vi "RT Driver VI.vi"(6 "Device Clock":string, 9 "Device Inputs FIFO":refnum<k33>, 10 "Device Outputs FIFO":refnum<k33>, 11 "Device Reference":T1 format="%.0x") -> ()   [LabVIEW 2015, in "Engine Simulation Toolkit Engine.lvlib"]
uses:
  Engine Simulation Toolkit Engine.lvlib
  <vilib>/NI Veristand/Custom Device API/Custom Device Item Ref.ctl
  <vilib>/Platform/TimedLoop/XDataNode/timing_clust.ctl
  <vilib>/Platform/TimedLoop/XDataNode/nitl_modes.ctl
  <vilib>/Platform/TimedLoop/XDataNode/wakeup.ctl
  Digital Pattern Gen 1.0 In Place Input Write Structure.vi
  APU 1.0 In Place Input Write Structure.vi
  APU 1.0 In Place Output Read Structure.vi
  Analog Replay 1.0 In Place Input Write Structure.vi
  Knock Cylinder 1.0 In Place Input Write Structure.vi
  Knock Sensor 1.0 In Place Input Write Structure.vi
  Directional Speed 1.0 In Place Input Write Structure.vi
  APU 1.1 In Place Input Write Structure.vi
  APU 1.1 In Place Output Read Structure.vi
  Digital Pattern Gen 1.3 In Place Input Write Structure.vi
  Digital Pattern Gen 1.3 In Place Settings Write Structure.vi
  APU 1.3 In Place Input Write Structure.vi
  APU 1.3 In Place Output Read Structure.vi
  Digital Pattern Gen 1.0 Write Inputs.vi
  APU 1.0 Write Inputs.vi
  Analog Replay 1.0 Voltage Scaling.vi
  Knock Cylinder 1.0 Write Inputs.vi
  Knock Sensor 1.0 Write Inputs.vi
  Directional Speed 1.0 Write Inputs.vi
  Digital Pattern Gen 1.3 Write Inputs.vi
  Digital Pattern Gen 1.3 Tooth to Edges.vi
  Shared/Angle in degrees to u16.vi
  Digital Pattern Gen 1.3 Validate Fault Positions.vi
  Shared/DBL Speed to FXP.vi
  Shared/Probability % to compare.vi
  Analog Replay 1.0 FPGA Inputs Write Node.vi
  Digital Pattern Gen 1.3 FPGA Settings Write Node.vi
  Digital Pattern Gen 1.0 FPGA Inputs Write Node.vi
  Knock Sensor 1.0 FPGA Inputs Write Node.vi
  Knock Cylinder 1.0 FPGA Inputs Write Node.vi
  Directional Speed 1.0 FPGA Inputs Write Node.vi
  Event Timing Capture 1.0 In Place Output Read Structure.vi
  Event Timing Measure 1.1 In Place Output Read Structure.vi
  Event Timing Measure 1.0 In Place Output Read Structure.vi
  APU 1.0 Read Outputs.vi
  APU 1.0 FPGA Inputs Write Node.vi
  <vilib>/Platform/TimedLoop/XDataNode/XDataNode.xnode
  <vilib>/NI Veristand/Custom Device Tools/Custom Device Utility Library/Custom Device Utility Library.lvlib
  <vilib>/Platform/TimedLoop/XDataNode/XDNodeRunTimeDep.lvlib
  <vilib>/NI Veristand/Custom Device API/Custom Device API.lvlib
panel:
  in  "Initialization Status Notifier":refnum<notifier>
  in  "Status Notifier":refnum<notifier>
  # "Custom Device Template\nv1.0"
  # "Use this template as a starting point for creating a custom device code module. The input controls shown here are specially named controls that the system will use to provide the device loop with data. The controls are not required for the device loop to run. For instance, if the device doesn't produce any output data, then you don't need the Device Outputs FIFO control. If you do use these controls, however, they need to have these exact names to be functional."
  # "The optional status notifier element is used to notify the RT engine of the last state of the custom device, and to indicate the device has completed execution. If this control is not used, a default No Error value is returned to the system when the device finishes execution.\n\nNote: This error state is not checked until the system shuts down. Use an output status channel to send more immediate status values to the system."
  # "This optional input can be used to send the VeriStand Engine the final status of the custom device initalization process. If this control exists on the custom device front panel, the VeriStand Engine will wait for a status update before starting up. If the custom device reports an error, that will abort the execution of the current configuration in the VeriStand Engine.\n\nThis control can be deleted if the custom device does not need to send the initialization status update."
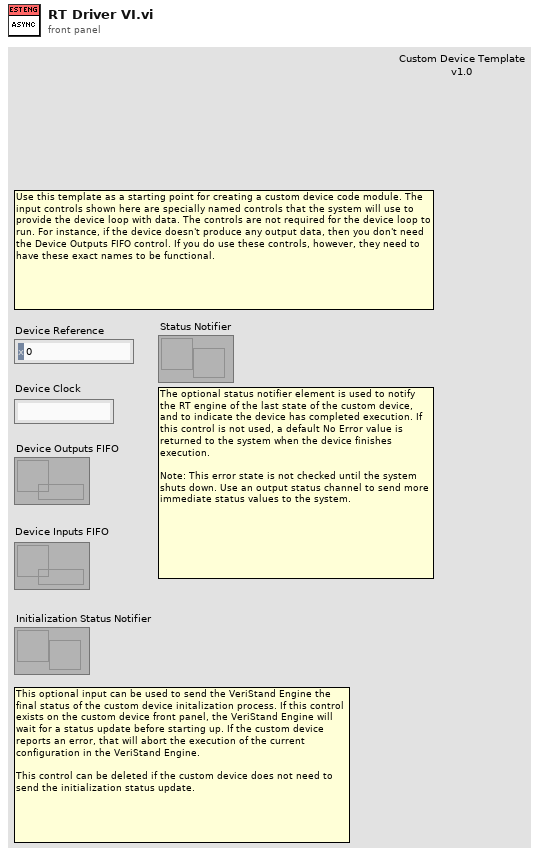
[diagram p1: front panel]
types:
  T1 = typedef "Custom Device API.lvlib/Custom Device Item Ref.ctl" = u64
  T2 = typedef "Engine Simulation Toolkit Engine.lvlib/RT Data.ctl" = cluster{"Compiled Data":T3, "FPGA Refs":T28}
  T3 = typedef "Engine Simulation Toolkit Shared.lvlib/Compiled Data.ctl" = cluster{"Init":T4, "1.0 APUs":T5[], "Status":T7, "DevOutFIFO":refnum<k33>, "DevInFIFO":refnum<k33>, "Device Inputs":dbl[], "Device Outputs":dbl[], "Last Device Inputs":dbl[], "1.0 Analog Replays":T8[], "Unused Analog Replays":string[], "1.0 Digital Pattern Gens":T10[], "Unused Digital Pattern Gens":string[], "1.0 Event Captures":T12[], "1.0 Event Measures":T14[], "1.0 Knock Sensors":T16[], "1.0 Knock Cylinders":T18[], "1.0 Directional Speed":T20[], "Unused Directional Sensors":string[], "1.1 APUs":T22[], "1.1 Event Measures":T23[], "1.3 Digital Pattern Gens":T24[], "Bitfile EST Version":T26, "1.3 APUs":T27[]}
  T4 = typedef "Engine Simulation Toolkit Shared.lvlib/Engine Init Data.ctl" = cluster{"CPU":i32, "RIO Address":string, "Decimation":i64, "Priority":i32, "Name":string, "Bitfile Path":path, "Input FIFO Size":i32, "Output FIFO Size":i32}
  T5 = typedef "Engine Simulation Toolkit Shared.lvlib/1.0 APU Engine Data.ctl" = cluster{"register names":cluster{"shared settings":string, "input":string, "settings":string, "output":string}, "shared settings":cluster{"cycle start":fxp<+,2,2>, "crank start":u16, "stuck limit":fxp<+,18,18>}, "settings":cluster{"acceleration":fxp<+,18,-20>, "max cycle":fxp<+,2,2>, "enable accel":bool}, "FIFO indexes":T6, "input":cluster{"desired speed":fxp<+/-,23,2>, "reset":bool}, "degrees of 1 cycle u16":dbl, "degrees of 1 crank u16":dbl}
  T6 = typedef "Engine Simulation Toolkit Shared.lvlib/1.0 APU Engine FIFO Idxs.ctl" = cluster{"inputs":cluster{"desired speed":i32, "reset":i32}, "outputs":cluster{"crank angle":i32, "cycle angle":i32, "actual speed":i32}}
  T7 = typedef "Engine Simulation Toolkit Shared.lvlib/Engine Status Data.ctl" = cluster{"FIFO indexes":cluster{"code":i32, "loop duration":i32, "late count":i32}}
  T8 = typedef "Engine Simulation Toolkit Shared.lvlib/1.0 Analog Replay Engine Data.ctl" = cluster{"register names":cluster{"load input":string, "settings":string, "input":string}, "settings":cluster{"ReverseNegate":bool, "CycleAngle":bool, "SpeedThreshold":fxp<+/-,23,2>, "AOBelowThreshold":i16}, "FIFO indexes":T9, "input":cluster{"Offset":i16, "VScaleSlope":fxp<+,18,6>, "VScaleIntercept":fxp<+/-,18,3>}, "offset convert":dbl, "DAC LUT":i16[], "SE_VScaleIntercept":fxp<+/-,18,3>, "SE_VScaleSlope":fxp<+,18,6>, "VOverride":bool, "ResetVolts":bool}
  T9 = typedef "Engine Simulation Toolkit Shared.lvlib/1.0 Analog Replay FIFO Idxs.ctl" = cluster{"enable voltage":i32, "volt slope":i32, "volt intercept":i32, "offset":i32}
  T10 = typedef "Engine Simulation Toolkit Shared.lvlib/1.0 Digital Pattern Gen Engine Data.ctl" = cluster{"register names":cluster{"load input":string, "settings":string, "input":string}, "settings":cluster{"edge 1":u16, "edge 2":u16, "cycle angle":bool, "enabled":bool, "first falling":bool}, "FIFO indexes":T11, "input":cluster{"Offset":i16}, "offset convert":dbl, "Position LUT":u16[]}
  T11 = typedef "Engine Simulation Toolkit Shared.lvlib/1.0 Digital Pattern Gen FIFO Idxs.ctl" = cluster{"offset":i32}
  T12 = typedef "Engine Simulation Toolkit Shared.lvlib/1.0 Event Timing Capture Engine Data.ctl" = cluster{"register names":cluster{"output":string}, "FIFO indexes":T13, "degrees of 1 u16":dbl, "wrap":bool, "window min":u16, "duration convert":dbl, "default start":dbl, "default end":dbl, "ref angle":dbl}
  T13 = typedef "Engine Simulation Toolkit Shared.lvlib/1.0 Event Timing Capture FIFO Idxs.ctl" = cluster{"start angle":i32, "end angle":i32, "duration":i32}
  T14 = typedef "Engine Simulation Toolkit Shared.lvlib/1.0 Event Timing Measure Engine Data.ctl" = cluster{"register names":cluster{"settings":string, "output":string}, "settings":cluster{"max":u16, "min":u16, "active high":bool, "wrap":bool, "full window":bool}, "FIFO indexes":T15}
  T15 = typedef "Engine Simulation Toolkit Shared.lvlib/1.0 Event Timing Measure FIFO Idxs.ctl" = cluster{"stuck active":i32, "win all active":i32, "win orph start":i32, "win orph end":i32}
  T16 = typedef "Engine Simulation Toolkit Shared.lvlib/1.0 Knock Sensor Engine Data.ctl" = cluster{"register names":cluster{"settings":string, "input":string}, "settings":cluster{"low freq (periods/tick)":fxp<+,32,0>, "high freq (periods/tick)":fxp<+,32,0>, "duration (1.25MHz tics)":fxp<+,18,18>, "low freq speed slope":fxp<+,16,-3>, "low freq speed intercept":fxp<+,10,-10>, "low freq by speed":bool}, "DAC multiplier":dbl, "FIFO indexes":T17, "input":cluster{"low freq scaler":fxp<+,10,0>}}
  T17 = typedef "Engine Simulation Toolkit Shared.lvlib/1.0 Knock Sensor FIFO Idxs.ctl" = cluster{"amp":i32}
  T18 = typedef "Engine Simulation Toolkit Shared.lvlib/1.0 Knock Cylinder Engine Data.ctl" = cluster{"register names":cluster{"settings":string, "input":string}, "settings":cluster{"seed":u16, "reset":bool}, "input":cluster{"probability compare":u16, "high freq scaler":fxp<+,10,0>, "trigger position":u16}, "DAC multiplier":dbl, "FIFO indexes":T19, "Angle multiplier":dbl}
  T19 = typedef "Engine Simulation Toolkit Shared.lvlib/1.0 Knock Cylinder FIFO Idxs.ctl" = cluster{"prob":i32, "amp":i32, "pos":i32}
  T20 = typedef "Engine Simulation Toolkit Shared.lvlib/1.0 Directional Speed Engine Data.ctl" = cluster{"register names":cluster{"settings":string, "input":string, "load input":string}, "settings":cluster{"Upper Value":u16, "Lower Value":u16, "Upper Index":fxp<+,10,10>, "Lower Index":fxp<+,10,10>, "Enabled":bool}, "input":cluster{"td (tics)":u16, "tf (tics)":u16, "tr (tics)":u16}, "FIFO indexes":T21, "Tooth Centers LUT":u16[]}
  T21 = typedef "Engine Simulation Toolkit Shared.lvlib/1.0 Directional Speed FIFO Idxs.ctl" = cluster{"td":i32, "tf":i32, "tr":i32}
  T22 = typedef "Engine Simulation Toolkit Shared.lvlib/1.1 APU Engine Data.ctl" = cluster{"register names":cluster{"shared settings":string, "input":string, "settings":string, "output":string, "go":string}, "shared settings":cluster{"cycle start":fxp<+,2,2>, "crank start":u16, "stuck limit":fxp<+,18,18>}, "settings":cluster{"acceleration":fxp<+,18,-20>, "max cycle":fxp<+,2,2>, "enable accel":bool}, "FIFO indexes":T6, "input":cluster{"desired speed":fxp<+/-,23,2>, "reset":bool}, "degrees of 1 cycle u16":dbl, "degrees of 1 crank u16":dbl}
  T23 = typedef "Engine Simulation Toolkit Shared.lvlib/1.1 Event Timing Measure Engine Data.ctl" = cluster{"register names":cluster{"settings":string, "output":string}, "settings":cluster{"max":u16, "min":u16, "active high":bool, "wrap":bool}, "FIFO indexes":T15}
  T24 = typedef "Engine Simulation Toolkit Shared.lvlib/1.3 Digital Pattern Gen Engine Data.ctl" = cluster{"register names":cluster{"load input":string, "settings":string, "input":string}, "settings":cluster{"edge 1":u16, "edge 2":u16, "cycle angle":bool, "enabled":bool, "first falling":bool, "fault":bool, "fault wrap":bool, "fault value":bool, "fault count":fxp<+,4,4>, "use fault count":bool}, "FIFO indexes":T25, "input":cluster{"Offset":i16}, "deg to u16 scale":dbl, "Position LUT":u16[], "# of teeth":i16, "max angle":dbl}
  T25 = typedef "Engine Simulation Toolkit Shared.lvlib/1.3 Digital Pattern Gen FIFO Idxs.ctl" = cluster{"offset":i32, "command":i32, "rotations":i32, "start angle":i32, "stop angle":i32, "tooth to rem":i32, "trigger":i32, "valid":i32}
  T26 = typedef "Engine Simulation Toolkit Shared.lvlib/Bitfile EST Version.ctl" = enum16{"1.0", "1.1", "1.2", "1.3"}
  T27 = typedef "Engine Simulation Toolkit Shared.lvlib/1.3 APU Engine Data.ctl" = cluster{"register names":cluster{"shared settings":string, "input":string, "settings":string, "output":string, "go":string}, "shared settings":cluster{"start":fxp<+,17,17>, "stuck limit":fxp<+,18,18>}, "settings":cluster{"acceleration":fxp<+,18,-20>, "enable accel":bool}, "FIFO indexes":T6, "input":cluster{"desired speed":fxp<+/-,23,2>, "reset":bool}, "degrees of 1 cycle u16":dbl, "degrees of 1 crank u16":dbl}
  T28 = typedef "Engine Simulation Toolkit Engine.lvlib/FPGA Refs.ctl" = cluster{"1.0 APUs":T29[], "FPGA ref":refnum<k20>, "1.0 Analog Replays":T32[], "1.0 Dig Pat Gens":T33[], "1.0 Event Captures":T34[], "1.0 Event Measures":T35[], "1.0 Knock Cylinders":T36[], "1.0 Knock Sensors":T37[], "1.0 Directional Speed Sensors":T38[], "1.3 Dig Pat Gens":T39[]}
  T29 = typedef "Engine Simulation Toolkit Engine.lvlib/APU 1.0 Run Refs.ctl" = cluster{"output reference":T30, "input reference":T31}
  T30 = typedef "Engine Simulation Toolkit Engine.lvlib/APU 1.0 Output Ref.ctl" = refnum<k20>
  T31 = typedef "Engine Simulation Toolkit Engine.lvlib/APU 1.0 Input Ref.ctl" = refnum<k20>
  T32 = typedef "Engine Simulation Toolkit Engine.lvlib/Analog Replay 1.0 Input Ref.ctl" = refnum<k20>
  T33 = typedef "Engine Simulation Toolkit Engine.lvlib/Digital Pattern Gen 1.0 Input Ref.ctl" = refnum<k20>
  T34 = typedef "Engine Simulation Toolkit Engine.lvlib/Event Timing Capture 1.0 Output Ref.ctl" = refnum<k20>
  T35 = typedef "Engine Simulation Toolkit Engine.lvlib/Event Timing Measure 1.0 Output Ref.ctl" = refnum<k20>
  T36 = typedef "Engine Simulation Toolkit Engine.lvlib/Knock Cylinder 1.0 Input Ref.ctl" = refnum<k20>
  T37 = typedef "Engine Simulation Toolkit Engine.lvlib/Knock Sensor 1.0 Input Ref.ctl" = refnum<k20>
  T38 = typedef "Engine Simulation Toolkit Engine.lvlib/Directional Speed 1.0 Input Ref.ctl" = refnum<k20>
  T39 = typedef "Engine Simulation Toolkit Engine.lvlib/Digital Pattern Gen 1.3 Run Refs.ctl" = cluster{"input":T33, "settings":T40}
  T40 = typedef "Engine Simulation Toolkit Engine.lvlib/Digital Pattern Gen 1.3 Settings Ref.ctl" = refnum<k20>
  T41 = typedef "XDNodeRunTimeDep.lvlib/timing_clust.ctl" = cluster{"Expected End [f-1]":u64, "Actual End [f-1]":u64, "Finished Late? [f-1]":bool, "Expected End [i-1]":u64, "Actual End [i-1]":u64, "Finished Late? [i-1]":bool, "Expected Start [i]":u64, "Actual Start [i]":u64, "Expected Start [f]":u64, "Actual Start [f]":u64, "Source Name":string, "Structure Name":string, "Period":i64, "Deadline":i64, "Offset":i64, "Start":i64, "Priority":i32, "Timeout":i32, "Mode":T42, "Wakeup Reason":T43, "Error":errorcluster, "Source Type":string, "Secondary Source Type":string, "Global End Time":u64, "Global Start Time":u64, "Frame Duration":u64, "Iteration Duration":u64, "Assigned CPU":i32, "I/O Scan Engine Mode":u32}
  T42 = typedef "XDNodeRunTimeDep.lvlib/nitl_modes.ctl" = enum32{"No Change", "Process missed periods, maintain original phase", "Discard missed periods, maintain original phase", "Process missed periods, ignore original phase", "Discard missed periods, ignore original phase"}
  T43 = typedef "XDNodeRunTimeDep.lvlib/wakeup.ctl" = enum32{"Normal", "Aborted", "Asynchronous wakeup", "Timing source error", "Timed loop error", "Timeout"}
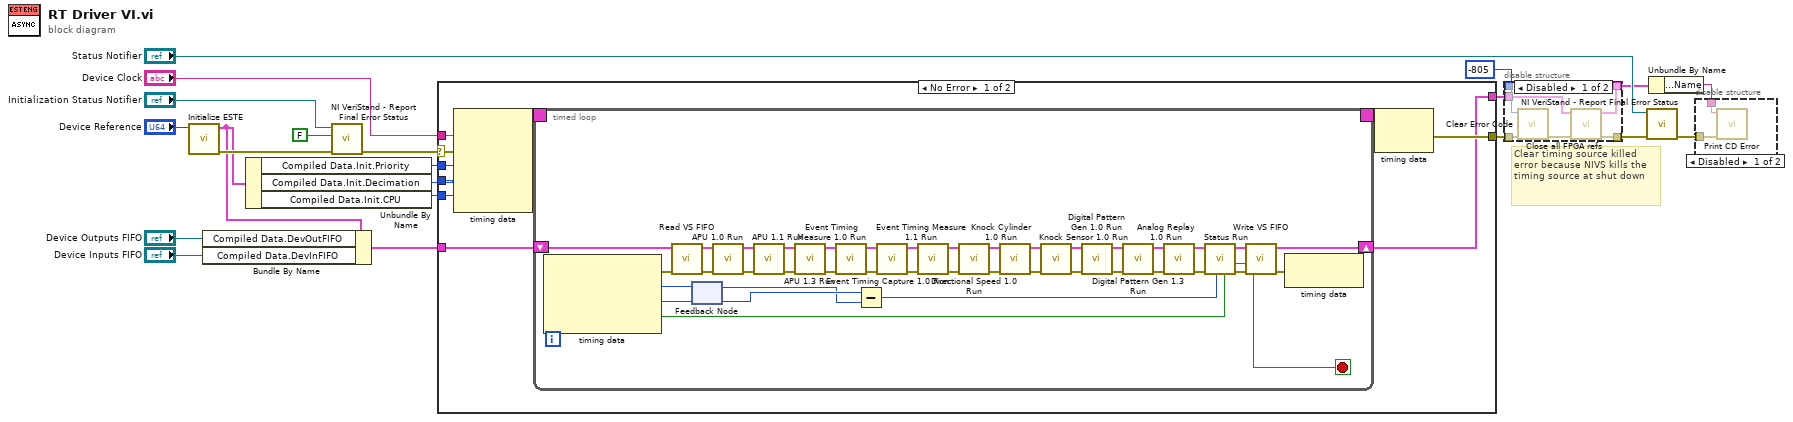
[diagram p0: block diagram]
diagram:
  # "Clear timing source killed error because NIVS kills the timing source at shut down"
  n1 = call "Initialize ESTE.vi"("Device Reference"="Device Reference") -> ("error out"=w21:errorcluster, "RT Data"=w12:T2)  [unwired: 9 in]
  n2 = Bundle By Name(cluster=w12, "Compiled Data.DevOutFIFO"="Device Outputs FIFO", "Compiled Data.DevInFIFO"="Device Inputs FIFO") -> (w3:T2)
  n3 = Unbundle By Name(w12) -> ("Compiled Data.Init.Priority"=w15:i32, "Compiled Data.Init.Decimation"=w14:i64, "Compiled Data.Init.CPU"=w13:i32)
  n4 = call <vilib>:"NI VeriStand - Report Final Error Status.vi"("error in (no error)"=w21, "Filter FIFO & Shutdown Errors (T)"=FALSE ("Filter FIFO Errors (T)"), "Status Notifier"="Initialization Status Notifier") -> ("error out"=w4:errorcluster)  [unwired: 8 out]
  n5 = case shown="No Error" w4 {
    selector: w4 -> [w28 w88]
    tunnel: [w29 w88] -> w1
    tunnel: "Device Clock" -> [w27 _]
    tunnel: w15 -> [w26 _]
    tunnel: w14 -> [w25 _]
    tunnel: w13 -> [w24 _]
    tunnel: w3 -> [w23 w87]
    tunnel: [w22 w87] -> w8
    frame No Error {
      n6 = node-c288(w27, w28, w26, w25, w24) -> (w31:T41)
      n7 = timed-loop {
        timing: w31 -> [_]
        timing-out: [_] -> w30
        shift-right: [w66] -> w22
        shift-left: w23 -> [w68]
        stop <- w64 stop-if-true
        n8 = node-c288() -> (w69:errorcluster, w63:i64, w62:i64, w65:bool)  [unwired: 1 in]
        n9 = call "Read VS FIFO.vi"("error in (no error)"=w69, "rt data in"=w68) -> ("error out"=w52:errorcluster, "rt data out"=w51:T2)  [unwired: 8 in]
        n10 = feedback #1() -> (w47:i64)  [unwired: 1 in]
        n11 = feedback-in #1(w63) -> ()
        n12 = call "APU 1.0 Run.vi"("error in (no error)"=w52, "rt data in"=w51) -> ("error out"=w58:errorcluster, "rt data out"=w41:T2)  [unwired: 8 in]
        n13 = call "APU 1.1 Run.vi"("error in (no error)"=w58, "rt data in"=w41) -> ("error out"=w42:errorcluster, "rt data out"=w33:T2)  [unwired: 8 in]
        n14 = call "APU 1.3 Run.vi"("error in (no error)"=w42, "rt data in"=w33) -> ("error out"=w34:errorcluster, "rt data out"=w32:T2)  [unwired: 8 in]
        n15 = call "Event Timing Measure 1.0 Run.vi"("error in (no error)"=w34, "rt data in"=w32) -> ("error out"=w57:errorcluster, "rt data out"=w39:T2)  [unwired: 8 in]
        n16 = Subtract(x=w62, y=w47) -> (x-y=w46:i64)
        n17 = call "Event Timing Measure 1.1 Run.vi"("error in (no error)"=w57, "rt data in"=w39) -> ("error out"=w40:errorcluster, "rt data out"=w38:T2)  [unwired: 8 in]
        n18 = call "Event Timing Capture 1.0 Run.vi"("error in (no error)"=w40, "rt data in"=w38) -> ("error out"=w60:errorcluster, "rt data out"=w44:T2)  [unwired: 8 in]
        n19 = call "Directional Speed 1.0 Run.vi"("error in (no error)"=w60, "rt data in"=w44) -> ("error out"=w45:errorcluster, "rt data out"=w43:T2)  [unwired: 8 in]
        n20 = call "Knock Cylinder 1.0 Run.vi"("error in (no error)"=w45, "rt data in"=w43) -> ("error out"=w56:errorcluster, "rt data out"=w54:T2)  [unwired: 8 in]
        n21 = call "Knock Sensor 1.0 Run.vi"("error in (no error)"=w56, "rt data in"=w54) -> ("error out"=w55:errorcluster, "rt data out"=w53:T2)  [unwired: 8 in]
        n22 = call "Digital Pattern Gen 1.0 Run.vi"("error in (no error)"=w55, "rt data in"=w53) -> ("error out"=w59:errorcluster, "rt data out"=w36:T2)  [unwired: 8 in]
        n23 = call "Digital Pattern Gen 1.3 Run.vi"("error in (no error)"=w59, "rt data in"=w36) -> ("error out"=w37:errorcluster, "rt data out"=w35:T2)  [unwired: 8 in]
        n24 = call "Analog Replay 1.0 Run.vi"("error in (no error)"=w37, "rt data in"=w35) -> ("error out"=w61:errorcluster, "rt data out"=w49:T2)  [unwired: 8 in]
        n25 = call "Status Run.vi"("Finished Late? [i-1]"=w65, "Iteration Duration"=w46, "error in (no error)"=w61, "rt data in"=w49) -> ("error out"=w50:errorcluster, "stop"=w64:bool, "rt data out"=w48:T2)  [unwired: 5 in]
        n26 = call "Write VS FIFO.vi"("error in (no error)"=w50, "compiled data in"=w48) -> ("error out"=w67:errorcluster, "compiled data out"=w66:T2)  [unwired: 8 in]
        n27 = node-c288(w67) -> ()  [unwired: 1 out]
      }
      n28 = node-c288(w30) -> (w29:errorcluster)
    }
    frame Error {
    }
  }
  n29 = disable-structure shown="Disabled" {
    disable-tunnel: [w94 _] -> w9
    disable-tunnel: w8 -> [w93 _]
    disable-tunnel: [w92 _] -> w7
    disable-tunnel: -805 ("y") -> [w91 _]
    disable-tunnel: w1 -> [w90 _]
    frame Disabled {
      n30 = call "Clear Error Code.vi"("error in (no error)"=w90, "Code"=w91) -> ("error out"=w89:errorcluster)  [unwired: 9 in]
      n31 = call "Close all FPGA refs.vi"("error in (no error)"=w89, "rt data in"=w93) -> ("error out"=w94:errorcluster, "rt data out"=w92:T2)  [unwired: 8 in]
    }
    frame Enabled {
    }
  }
  n32 = call <vilib>:"NI VeriStand - Report Final Error Status.vi"("error in (no error)"=w9, "Status Notifier"="Status Notifier") -> ("error out"=w6:errorcluster)  [unwired: 1 in, 8 out]
  n33 = Unbundle By Name(w7) -> ("Compiled Data.Init.Name"=w5:string)
  n34 = disable-structure shown="Disabled" {
    disable-tunnel: w6 -> [w96 _]
    disable-tunnel: w5 -> [w95 _]
    frame Disabled {
      n35 = call "Print CD Error.vi"("error in"=w96, "Your code's public name"=w95) -> ()  [unwired: 8 in, 1 out]
    }
    frame Enabled {
    }
  }
